vi "DOE Show Events.vi"(5 "Flow Rate":dbl, 6 "Data Logger Type":T1=enum."Agilent", 7 "Agilent Digital Events":bool[](array[boolean]), 8 "Error In":errorcluster, 10 "Data Input":dbl[](array[numeric]), 11 "Kitchen Cluster Inlet":T2) -> (0 "Error Out":errorcluster, 3 "Kitchen Cluster Output":T2, 4 "sorted array":i32[](array[numeric]))   [LabVIEW 2019]
uses:
  Type Definitions/DOE Kitchen Control.ctl
  Type Definitions/DOE Data Logger Type.ctl
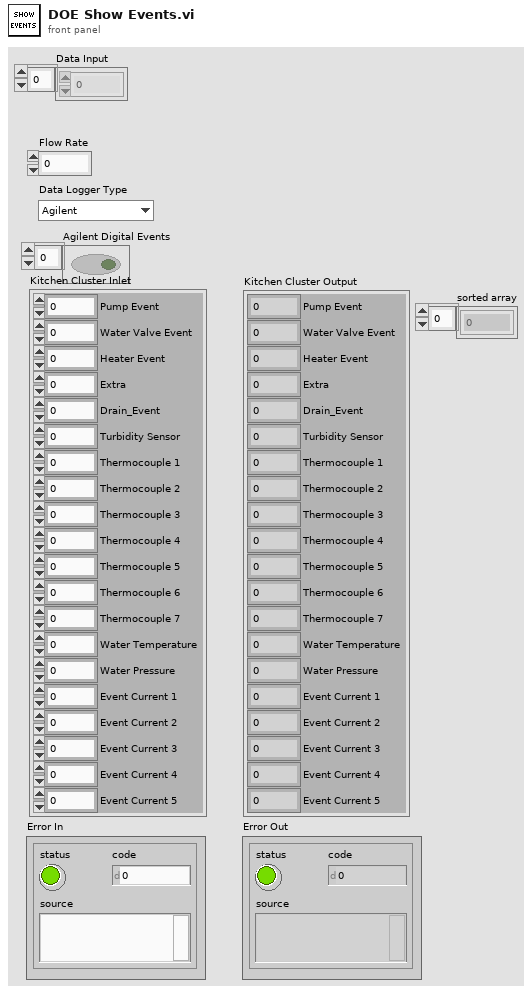
[diagram p1: front panel]
types:
  T1 = typedef "DOE Data Logger Type.ctl" = enum16{"MW100", "Agilent", "Agilent_Laurel_DC_Clamp"}
  T2 = typedef "DOE Kitchen Control.ctl" = cluster{"Drain_Event":i16, "Pump Event":i16, "Water Valve Event":i16, "Heater Event":i16, "Extra":i16, "Turbidity Sensor":dbl, "Thermocouple 1":dbl, "Thermocouple 2":dbl, "Thermocouple 3":dbl, "Thermocouple 4":dbl, "Thermocouple 5":dbl, "Thermocouple 6":dbl, "Water Temperature":dbl, "Water Pressure":dbl, "Event Current 1":dbl, "Event Current 2":dbl, "Event Current 3":dbl, "Event Current 4":dbl, "Event Current 5":dbl, "Thermocouple 7":dbl}
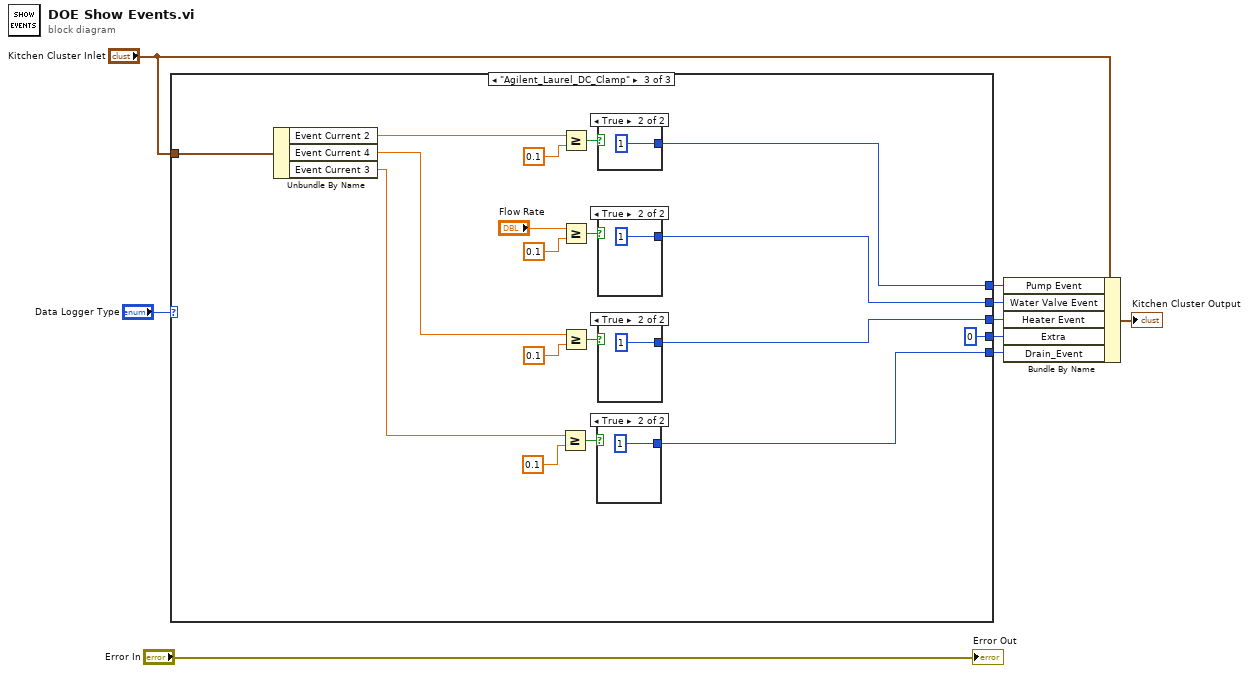
[diagram p0: block diagram]
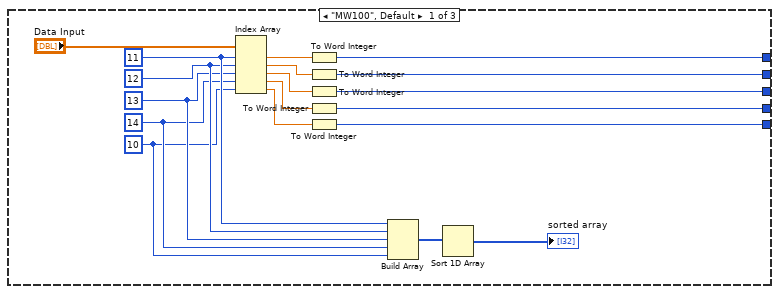
[diagram p2: hidden frame]
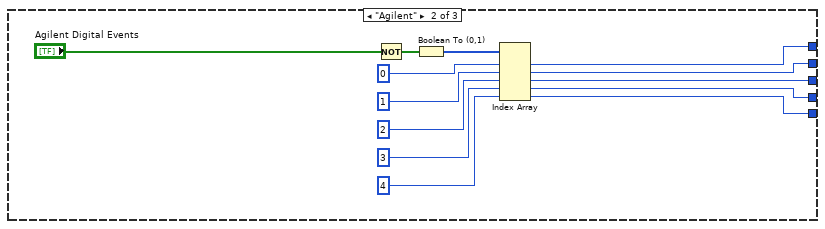
[diagram p3: hidden frame]
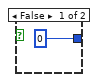
[diagram p4: hidden frame]
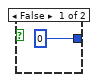
[diagram p5: hidden frame]
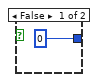
[diagram p6: hidden frame]
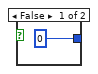
[diagram p7: hidden frame]
diagram:
  n1 = case shown="\"Agilent_Laurel_DC_Clamp\"" "Data Logger Type" {
    tunnel: [w26 w37 w56] -> w2
    tunnel: [w24 w36 w49] -> w8
    tunnel: [w22 w35 w48] -> w7
    tunnel: [w20 w34 i16 0 ("index")] -> w6
    tunnel: [w18 w33 w47] -> w4
    tunnel: "Kitchen Cluster Inlet" -> [_ _ w46]
    frame "MW100", Default {
      w12 = 10 ("index")
      w13 = 14 ("index")
      w14 = 13 ("index")
      w15 = 12 ("index")
      w16 = 11 ("index")
      n2 = Index Array(array="Data Input", index #1=w16, index #2=w15, index #3=w14, index #4=w13, index #5=w12) -> (element #1=w27:dbl, element #2=w25:dbl, element #3=w23:dbl, element #4=w21:dbl, element #5=w19:dbl)
      n3 = To Word Integer(number=w27) -> (16bit integer=w26:i16)
      n4 = To Word Integer(number=w25) -> (16bit integer=w24:i16)
      n5 = To Word Integer(number=w23) -> (16bit integer=w22:i16)
      n6 = To Word Integer(number=w21) -> (16bit integer=w20:i16)
      n7 = To Word Integer(number=w19) -> (16bit integer=w18:i16)
      n8 = Build Array(w16, w15, w14, w13, w12) -> (w11:i32[])
      n9 = Sort 1D Array(array=w11) -> (sorted array=→"sorted array":i32[])
    }
    frame "Agilent" {
      n10 = Not(x="Agilent Digital Events") -> (.not. x?=w40:bool[])
      n11 = Boolean To (0,1)(Boolean=w40) -> (0, 1=w39:i16[])
      n12 = Index Array(array=w39, index #1=0 ("index"), index #2=1 ("index"), index #3=2 ("index"), index #4=3 ("index"), index #5=4 ("index")) -> (element #1=w37:i16, element #2=w36:i16, element #3=w35:i16, element #4=w34:i16, element #5=w33:i16)
    }
    frame "Agilent_Laurel_DC_Clamp" {
      n13 = Unbundle By Name(w46) -> ("Event Current 2"=w45:dbl, "Event Current 4"=w44:dbl, "Event Current 3"=w43:dbl)
      n14 = Greater Or Equal?(x=w43, y=0.1) -> (x >= y?=w51:bool)
      n15 = Greater Or Equal?(x=w45, y=0.1) -> (x >= y?=w58:bool)
      n16 = Greater Or Equal?(x="Flow Rate", y=0.1) -> (x >= y?=w54:bool)
      n17 = Greater Or Equal?(x=w44, y=0.1) -> (x >= y?=w53:bool)
      n18 = case shown="True" w51 {
        tunnel: [i16 0 ("index") i16 1 ("index")] -> w47
        frame False {
        }
        frame True {
        }
      }
      n19 = case shown="True" w58 {
        tunnel: [i16 0 ("index") i16 1 ("index")] -> w56
        frame False {
        }
        frame True {
        }
      }
      n20 = case shown="True" w54 {
        tunnel: [i16 0 ("index") i16 1 ("index")] -> w49
        frame False {
        }
        frame True {
        }
      }
      n21 = case shown="True" w53 {
        tunnel: [i16 0 ("index") i16 1 ("index")] -> w48
        frame False {
        }
        frame True {
        }
      }
    }
  }
  n22 = Bundle By Name(cluster="Kitchen Cluster Inlet", "Pump Event"=w2, "Water Valve Event"=w8, "Heater Event"=w7, "Extra"=w6, "Drain_Event"=w4) -> (→"Kitchen Cluster Output":T2)
  "Error Out" <- "Error In"
